vi "Datasheet Histogram.vi"(6 "Connection Refnum":T2, 8 "error in (no error)":errorcluster, 9 "Grouped Results":cluster{"Result Group":T1[]}[](array[cluster]), 10 "sxTemplateId":string, 11 "Parameters":T3) -> (0 "error out":errorcluster, 3 "report":path)   [LabVIEW 2011]
uses:
  ITK EXT/utils/keyedarr.llb/Keyed Array.ctl
  Summitek EXT/ODBC/SQL Controls/Connection Refnum.ctl
  www/cgi-bin/_cgi-lib/TDM_INDEX Record.ctl
  ITK EXT/utils/strutil.llb/Case Matching.ctl
  Datasheet Analysis Parameters.ctl
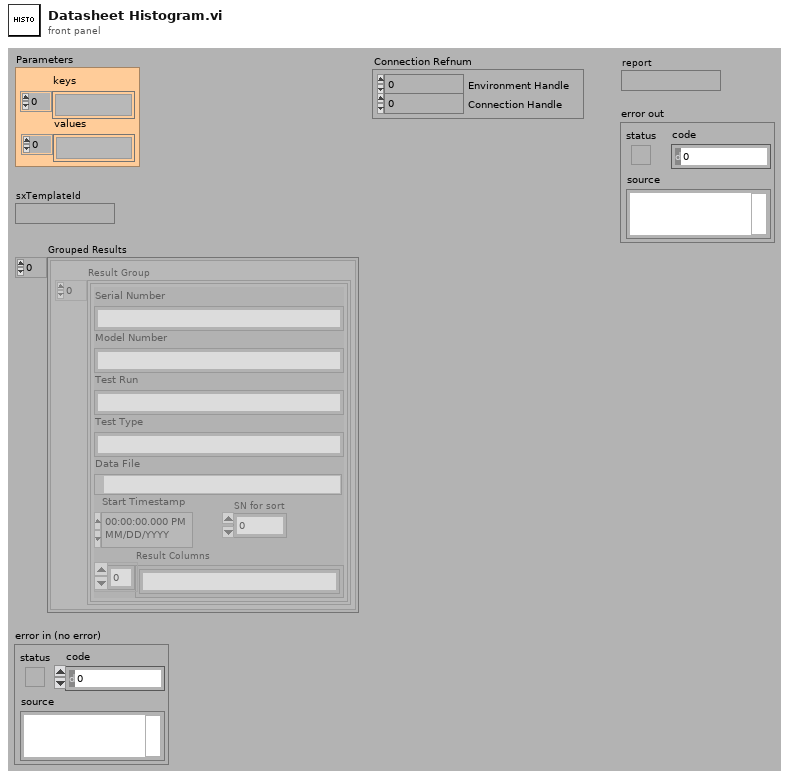
[diagram p1: front panel]
types:
  T1 = typedef "TDM_INDEX Record.ctl" = cluster{"Model Number":string, "SN for sort":i32, "Test Type":string, "Test Run":string, "Serial Number":string, "Start Timestamp":timestamp, "Data File":path, "Result Columns":string[]}
  T2 = typedef "Connection Refnum.ctl" = cluster{"Environment Handle":i32, "Connection Handle":i32}
  T3 = typedef "Keyed Array.ctl" = cluster{"keys":string[], "values":string[]}
  T4 = typedef "Datasheet Analysis Parameters.ctl" = cluster{"Test Type":string, "Parameter":string, "Sxx Format":string, "PIM Unit":string, "Start Frequency":dbl, "Stop Frequency":dbl, "Sort Property":string, "Show Raw?":bool, "Bin format":string, "Bin Type":string, "Bin_var":string}
  T5 = typedef "Case Matching.ctl" = enum16{"a != A", "a == A", "system"}
  T6 = typedef "Statistics Data.ctl" = cluster{"Table":T7[], "Frequencies":dbl[]}
  T7 = typedef "CGI SimpleStat Results.ctl" = cluster{"Model Number":string, "Serial Number for Sort":i32, "Serial Number":string, "Time Stamp":timestamp, "Channel Data":dbl[], "Test Status":string, "OperatorID":string, "Frequency Data":dbl[], "RunID":string, "Sort Property Value":string}
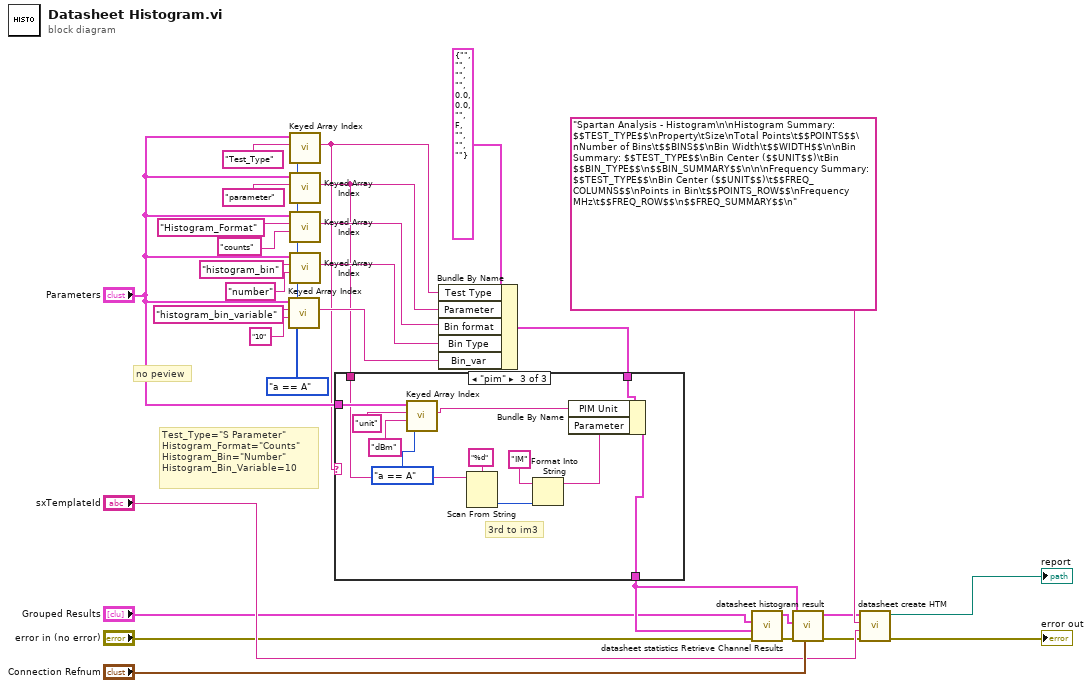
[diagram p0: block diagram]
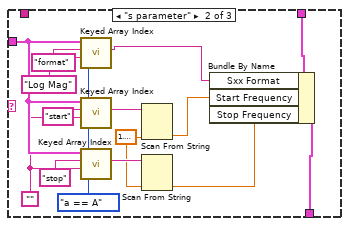
[diagram p3: hidden frame]
diagram:
  w24 = Case_Matching."a == A" ("case matching (sensitive)")
  # "no peview"
  # "Test_Type=\"S Parameter\"\nHistogram_Format=\"Counts\"\nHistogram_Bin=\"Number\"\nHistogram_Bin_Variable=10"
  n1 = call "Keyed Array Index.vi"("case matching (sensitive)"=w24, "default value"="10" ("format string"), "key"="histogram_bin_variable" ("format string"), "array in"="Parameters") -> ("value"=w26:string)  [unwired: 3 out]
  n2 = call "Keyed Array Index.vi"("case matching (sensitive)"=w24, "key"="Test_Type" ("format string"), "array in"="Parameters") -> ("value"=w10:string)  [unwired: 1 in, 3 out]
  n3 = call "Keyed Array Index.vi"("case matching (sensitive)"=w24, "key"="parameter" ("format string"), "array in"="Parameters") -> ("value"=w1:string)  [unwired: 1 in, 3 out]
  n4 = call "Keyed Array Index.vi"("case matching (sensitive)"=w24, "default value"="counts" ("format string"), "key"="Histogram_Format" ("format string"), "array in"="Parameters") -> ("value"=w6:string)  [unwired: 3 out]
  n5 = call "Keyed Array Index.vi"("case matching (sensitive)"=w24, "default value"="number" ("format string"), "key"="histogram_bin" ("format string"), "array in"="Parameters") -> ("value"=w25:string)  [unwired: 3 out]
  n6 = Bundle By Name(cluster=T4 {"Test Type"="", "Parameter"="", "Sxx Format"="", "PIM Unit"="", "Start Frequency"=0.0, "Stop Frequency"=0.0, "Sort Property"="", "Show Raw?"=FALSE, "Bin format"="", "Bin Type"="", "Bin_var"=""} ("Test Parameters"), "Test Type"=w10, "Parameter"=w1, "Bin format"=w6, "Bin Type"=w25, "Bin_var"=w26) -> (w11:T4)
  n7 = case shown="\"pim\"" w10 {
    tunnel: "Parameters" -> [_ w43 w57]
    tunnel: w11 -> [w30 w42 w56]
    tunnel: [w30 w41 w55] -> w13
    tunnel: w1 -> [_ _ w46]
    frame Default {
    }
    frame "s parameter" {
      w40 = Case_Matching."a == A" ("case matching (sensitive)")
      w32 = 1.1447298858494002
      w37 = ""
      n8 = call "Keyed Array Index.vi"("case matching (sensitive)"=w40, "default value"="Log Mag" ("format string"), "key"="format" ("format string"), "array in"=w43) -> ("value"=w39:string)  [unwired: 3 out]
      n9 = call "Keyed Array Index.vi"("case matching (sensitive)"=w40, "default value"=w37, "key"="start" ("format string"), "array in"=w43) -> ("value"=w35:string)  [unwired: 3 out]
      n10 = call "Keyed Array Index.vi"("case matching (sensitive)"=w40, "default value"=w37, "key"="stop" ("format string"), "array in"=w43) -> ("value"=w33:string)  [unwired: 3 out]
      n11 = Scan From String(input string=w35, default 1=w32) -> (output 1=w34:dbl)  [unwired: 3 in, 3 out]
      n12 = Scan From String(input string=w33, default 1=w32) -> (output 1=w31:dbl)  [unwired: 3 in, 3 out]
      n13 = Bundle By Name(cluster=w42, "Sxx Format"=w39, "Start Frequency"=w34, "Stop Frequency"=w31) -> (w41:T4)
    }
    frame "pim" {
      # "3rd to im3"
      n14 = call "Keyed Array Index.vi"("case matching (sensitive)"=Case_Matching."a == A", "default value"="dBm" ("format string"), "key"="unit" ("format string"), "array in"=w57) -> ("value"=w54:string)  [unwired: 3 out]
      n15 = Scan From String(format string="%d", input string=w46) -> (output 1=w49:i32)  [unwired: 2 in, 4 out]
      n16 = Format Into String(initial string="IM" ("format string"), w49) -> (resulting string=w47:string)  [unwired: 2 in, 1 out]
      n17 = Bundle By Name(cluster=w56, "PIM Unit"=w54, "Parameter"=w47) -> (w55:T4)
    }
  }
  n18 = call "datasheet statistics Retrieve Channel Results.vi"("error in (no error)"="error in (no error)", "Test Parameters"=w13, "Grouped Results"="Grouped Results") -> ("error out"=w12:errorcluster, "Stat Data"=w14:T6)  [unwired: 1 in, 6 out]
  n19 = call "datasheet histogram result.vi"("Connection Refnum"="Connection Refnum", "error in (no error)"=w12, "Histogram Results"=w14, "Query Parameters"=w13) -> ("error out"=w17:errorcluster, "Key Array"=w27:T3)  [unwired: 6 out]
  n20 = call "datasheet create HTM.vi"("error in (no error)"=w17, "sxTemplateId"="sxTemplateId", "template"="Spartan Analysis - Histogram\n\nHistogram Summary: $$TEST_TYPE$$\nProperty\tSize\nTotal Points\t$$POINTS$$\nNumber of Bins\t$$BINS$$\nBin Width\t$$WIDTH$$\n\nBin Summary: $$TEST_TYPE$$\nBin Center ($$UNIT$$)\tBin $$BIN_TYPE$$\n$$BIN_SUMMARY$$\n\n\nFrequency Summary: $$TEST_TYPE$$\nBin Center ($$UNIT$$)\t$$FREQ_COLUMNS$$\nPoints in Bin\t$$POINTS_ROW$$\nFrequency MHz\t$$FREQ_ROW$$\n$$FREQ_SUMMARY$$\n", "array out"=w27) -> ("error out"=→"error out":errorcluster, "report"=→"report":path)  [unwired: 6 out]
